vi "StageClose.vi"(8 "error in (no error)":errorcluster, 11 "StageHandle In":T1) -> (0 "error out":errorcluster)   [LabVIEW 2014]
doc: "Close the stage control"
uses:
  C:/Users/light/Desktop/SI+Raman/Labview/Raman/dll/Thorlabs.MotionControl.Controls.dll
  dll/Thorlabs.MotionControl.Controls.dll
  TypeDef/StageHandleOut.ctl
panel:
  # "Close the stage control"
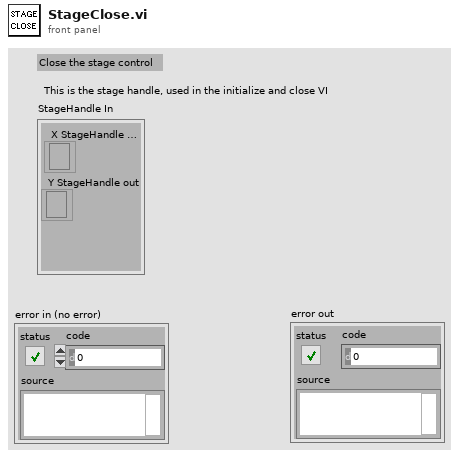
[diagram p1: front panel]
types:
  T1 = typedef "StageHandleOut.ctl" = cluster{"X StageHandle out":refnum<k24>, "Y StageHandle out":refnum<k24>}
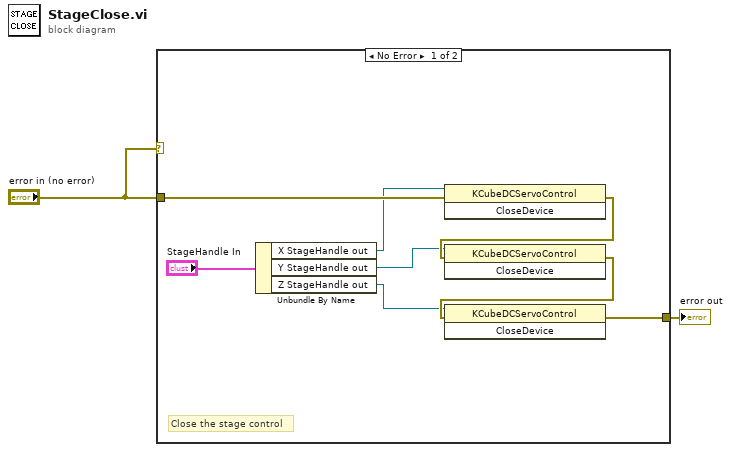
[diagram p0: block diagram]
diagram:
  n1 = case shown="No Error" "error in (no error)" {
    tunnel: "error in (no error)" -> [w10 w11]
    tunnel: [w7 w11] -> w1
    frame No Error {
      # "Close the stage control"
      n2 = Unbundle By Name("StageHandle In") -> ("X StageHandle out"=w5:refnum<k24>, "Y StageHandle out"=w4:refnum<k24>, "Z StageHandle out"=w3:refnum<k24>)
      n3 = invoke class="KCubeDCServoControl" method="CloseDevice"(reference=w5, error in=w10) -> (error out=w9:errorcluster)  [unwired: 1 in, 2 out]
      n4 = invoke class="KCubeDCServoControl" method="CloseDevice"(reference=w4, error in=w9) -> (error out=w8:errorcluster)  [unwired: 1 in, 2 out]
      n5 = invoke class="KCubeDCServoControl" method="CloseDevice"(reference=w3, error in=w8) -> (error out=w7:errorcluster)  [unwired: 1 in, 2 out]
    }
    frame Error {
    }
  }
  "error out" <- w1
